vi "Tenney Simulated Data.vi"(8 "error in (no error)":errorcluster, 10 "Tenney Environmental Chamber Data Input":T1) -> (0 "error out":errorcluster, 2 "Tenney Environmental Chamber Data Output":T1)   [LabVIEW 2023]
uses:
  Drivers/Tidal Engineering/Type Definitions/Tenney Environmental Chamber Data.ctl
  <vilib>/numeric/Random Number (Range) DBL.vi
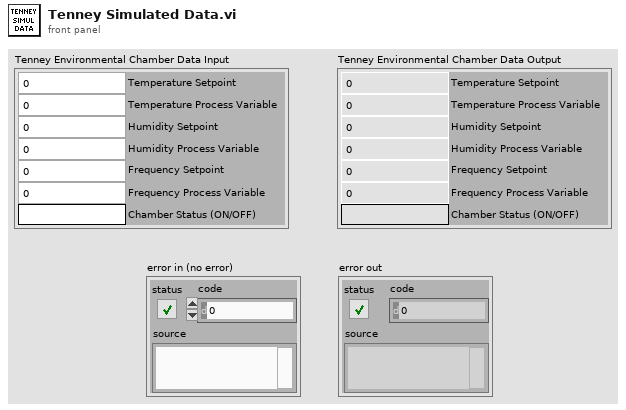
[diagram p1: front panel]
types:
  T1 = typedef "Tenney Environmental Chamber Data.ctl" = cluster{"Temperature Setpoint":dbl, "Temperature Process Variable":dbl, "Humidity Setpoint":dbl, "Humidity Process Variable":dbl, "Frequency Setpoint":dbl, "Frequency Process Variable":dbl, "Chamber Status (ON/OFF)":string}
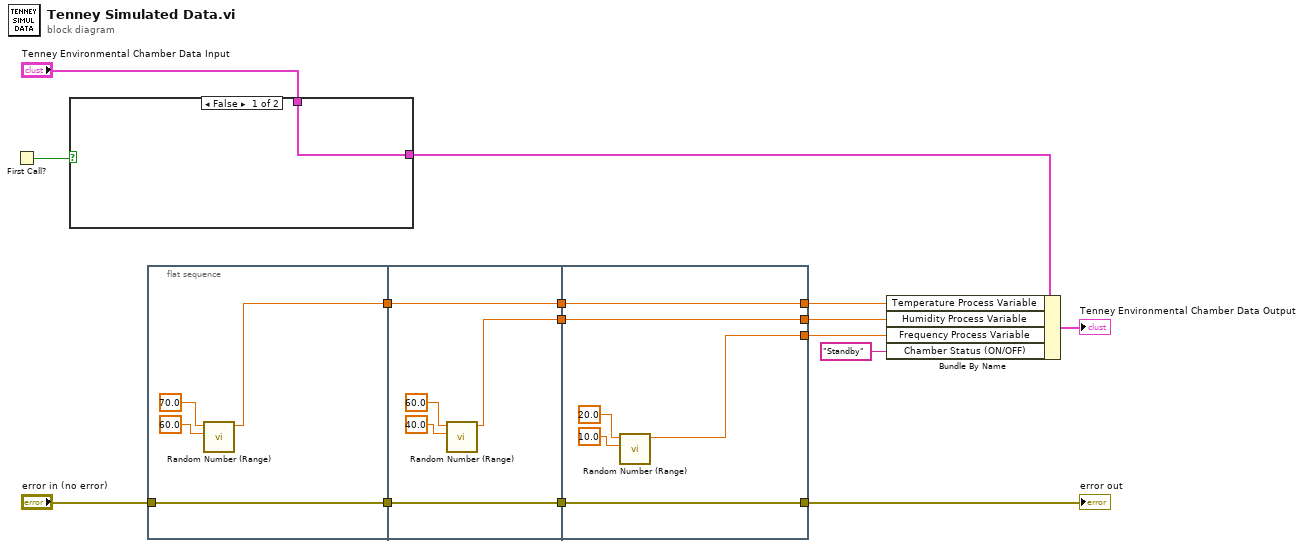
[diagram p0: block diagram]
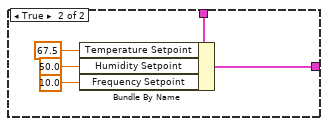
[diagram p2: hidden frame]
diagram:
  n1 = First Call?() -> (First Call?: T/F=w1:bool)
  n2 = case shown="False" w1 {
    tunnel: "Tenney Environmental Chamber Data Input" -> [w16 w21]
    tunnel: [w16 w20] -> w2
    frame False {
    }
    frame True {
      n3 = Bundle By Name(cluster=w21, "Temperature Setpoint"=67.5 ("upper bound (100)"), "Humidity Setpoint"=50.0 ("upper bound (100)"), "Frequency Setpoint"=10.0 ("lower bound (0)")) -> (w20:T1)
    }
  }
  n4 = flat-sequence {
    tunnel: "error in (no error)" -> [w23]
    tunnel: [w23] -> w15
    tunnel: [w22] -> w11
    tunnel: w15 -> [w30]
    tunnel: [w30] -> w14
    tunnel: w11 -> [w27]
    tunnel: [w27] -> w10
    tunnel: [w26] -> w8
    tunnel: [w36] -> w13
    tunnel: w14 -> [w36]
    tunnel: w10 -> [w33]
    tunnel: [w33] -> w9
    tunnel: [w32] -> w7
    tunnel: w8 -> [w32]
    tunnel: [w31] -> w6
    frame #0 {
      n5 = call-poly <vilib>:"Random Number (Range).vi"("lower bound (0)"=60.0, "upper bound (100)"=70.0) -> ("number"=w22:dbl)  [unwired: 9 in]
    }
    frame #1 {
      n6 = call-poly <vilib>:"Random Number (Range).vi"("lower bound (0)"=40.0, "upper bound (100)"=60.0) -> ("number"=w26:dbl)  [unwired: 9 in]
    }
    frame #2 {
      n7 = call-poly <vilib>:"Random Number (Range).vi"("lower bound (0)"=10.0, "upper bound (100)"=20.0) -> ("number"=w31:dbl)  [unwired: 9 in]
    }
  }
  n8 = Bundle By Name(cluster=w2, "Temperature Process Variable"=w9, "Humidity Process Variable"=w7, "Frequency Process Variable"=w6, "Chamber Status (ON/OFF)"="Standby") -> (→"Tenney Environmental Chamber Data Output":T1)
  "error out" <- w13
